vi "CFS-Compute Cal Transfer Function.vi"(0 "Mag":dbl[][](array[numeric]), 1 "Stimulus":dbl[](array[numeric]), 2 "Accel Gain (dB)":dbl=50000.0, 5 "Phase":dbl[][](array[numeric]), 7 "df (Hz)":dbl, 9 "Accelerometer Sens (mV/g)":dbl=50000.0, 11 "error in (no error)":errorcluster, 12 "Attenuation (dB)":dbl) -> (4 "Mag":dbl[](array[numeric]), 6 "Phase":dbl[](array[numeric]), 8 "Frequency":dbl[](array[numeric]), 15 "error out":errorcluster)   [LabVIEW 2015]
uses:
  Utility VIs/Math VIs/LinSpace (x0-dx-npts).vi
  Utility VIs/Math VIs/Linear to dB (scalar).vi
  Utility VIs/Math VIs/FFT x(t) to dB,Degrees (1D).vi
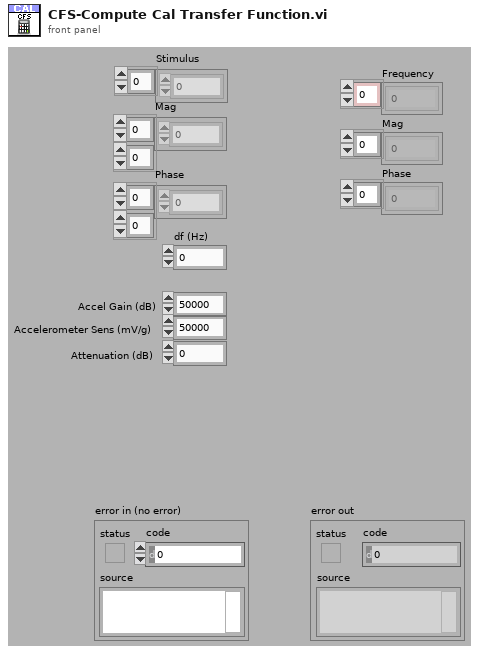
[diagram p1: front panel]
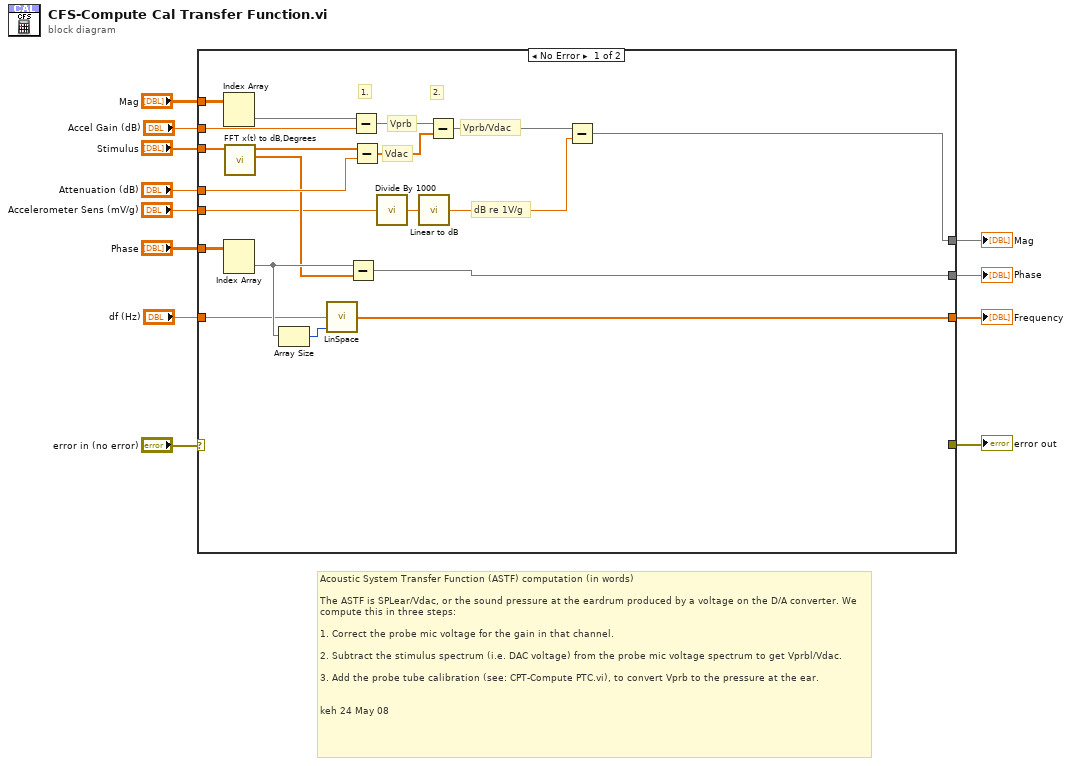
[diagram p0: block diagram]
diagram:
  # "Acoustic System Transfer Function (ASTF) computation (in words)\n\nThe ASTF is SPLear/Vdac, or the sound pressure at the eardrum produced by a voltage on the D/A converter. We compute this in three steps:\n\n1. Correct the probe mic voltage for the gain in that channel.\n\n2. Subtract the stimulus spectrum (i.e. DAC voltage) from the probe mic voltage spectrum to get Vprbl/Vdac.\n\n3. Add the probe tube calibration (see: CPT-Compute PTC.vi), to convert Vprb to the pressure at the ear.\n\n\nkeh 24 May 08"
  n1 = case shown="No Error" "error in (no error)" {
    selector: "error in (no error)" -> [_ w33]
    tunnel: "Mag" -> [w32 _]
    tunnel: "Phase" -> [w31 _]
    tunnel: [w14 _] -> w3
    tunnel: [w28 _] -> w10
    tunnel: "Stimulus" -> [w22 _]
    tunnel: "df (Hz)" -> [w18 _]
    tunnel: [w19 _] -> w6
    tunnel: "Accel Gain (dB)" -> [w26 _]
    tunnel: [_ w33] -> w5
    tunnel: "Attenuation (dB)" -> [w23 _]
    tunnel: "Accelerometer Sens (mV/g)" -> [w16 _]
    frame No Error {
      # "dB re 1V/g"
      # "2."
      # "1."
      # "Vprb/Vdac"
      # "Vdac"
      # "Vprb"
      n2 = Index Array(array=w32) -> (element=w25:dbl[])  [unwired: 2 in]
      n3 = Index Array(array=w31) -> (element=w30:dbl[])  [unwired: 2 in]
      n4 = call-poly "FFT x(t) to dB,Degrees.vi"("X"=w22) -> ("+Freq Phase of FFT (degrees)"=w17:dbl[], "+Freq. Mag of FFT (dB rms)"=w20:dbl[])  [unwired: 8 in, 1 out]
      n5 = Array Size(array=w30) -> (size(s)=w29:i32)
      n6 = call-poly "LinSpace.vi"("npts"=w29, "dx"=w18) -> ("Array"=w19:dbl[])  [unwired: 2 in, 1 out]
      n7 = Subtract(x=w30, y=w17) -> (x-y=w28:dbl[])
      n8 = Subtract(x=w25, y=w26) -> (x-y=w27:dbl[])
      n9 = Subtract(x=w20, y=w23) -> (x-y=w21:dbl[])
      n10 = call "Divide By 1000.vi"("X"=w16) -> ("X/1000"=w15:dbl)
      n11 = call-poly "Linear to dB.vi"("Linear"=w15) -> ("dB"=w13:dbl)
      n12 = Subtract(x=w27, y=w21) -> (x-y=w24:dbl[])
      n13 = Subtract(x=w24, y=w13) -> (x-y=w14:dbl[])
    }
    frame Error {
    }
  }
  "Mag" <- w3
  "Phase" <- w10
  "error out" <- w5
  "Frequency" <- w6
